vi "load pid.vi"(8 "error in (no error)":errorcluster, 11 "main ref":T1) -> (0 "error out":errorcluster)   [LabVIEW 2025]
uses:
  controls/LAB-IQ UI Data.ctl
  <vilib>/Analysis/baseanly.llb/Mean (DBL).vi
  <vilib>/Utility/error.llb/Trim Whitespace One-Sided.vi
  Instance           5 16Saved   load pid .vi
  <vilib>/Analysis/NI_AALBase.lvlib
  <vilib>/addons/control/pid/NI_PID_autopid.lvlib
panel:
  in  "WriteCC1":string[](array[string])=[""]
  out "apply load 2":bool
  out "Load":dbl
  out "Load Feedback":dbl
  out "Set Load 2":dbl=455.0
  out "Motorised Loading Loop":i32
  out "Zload":dbl
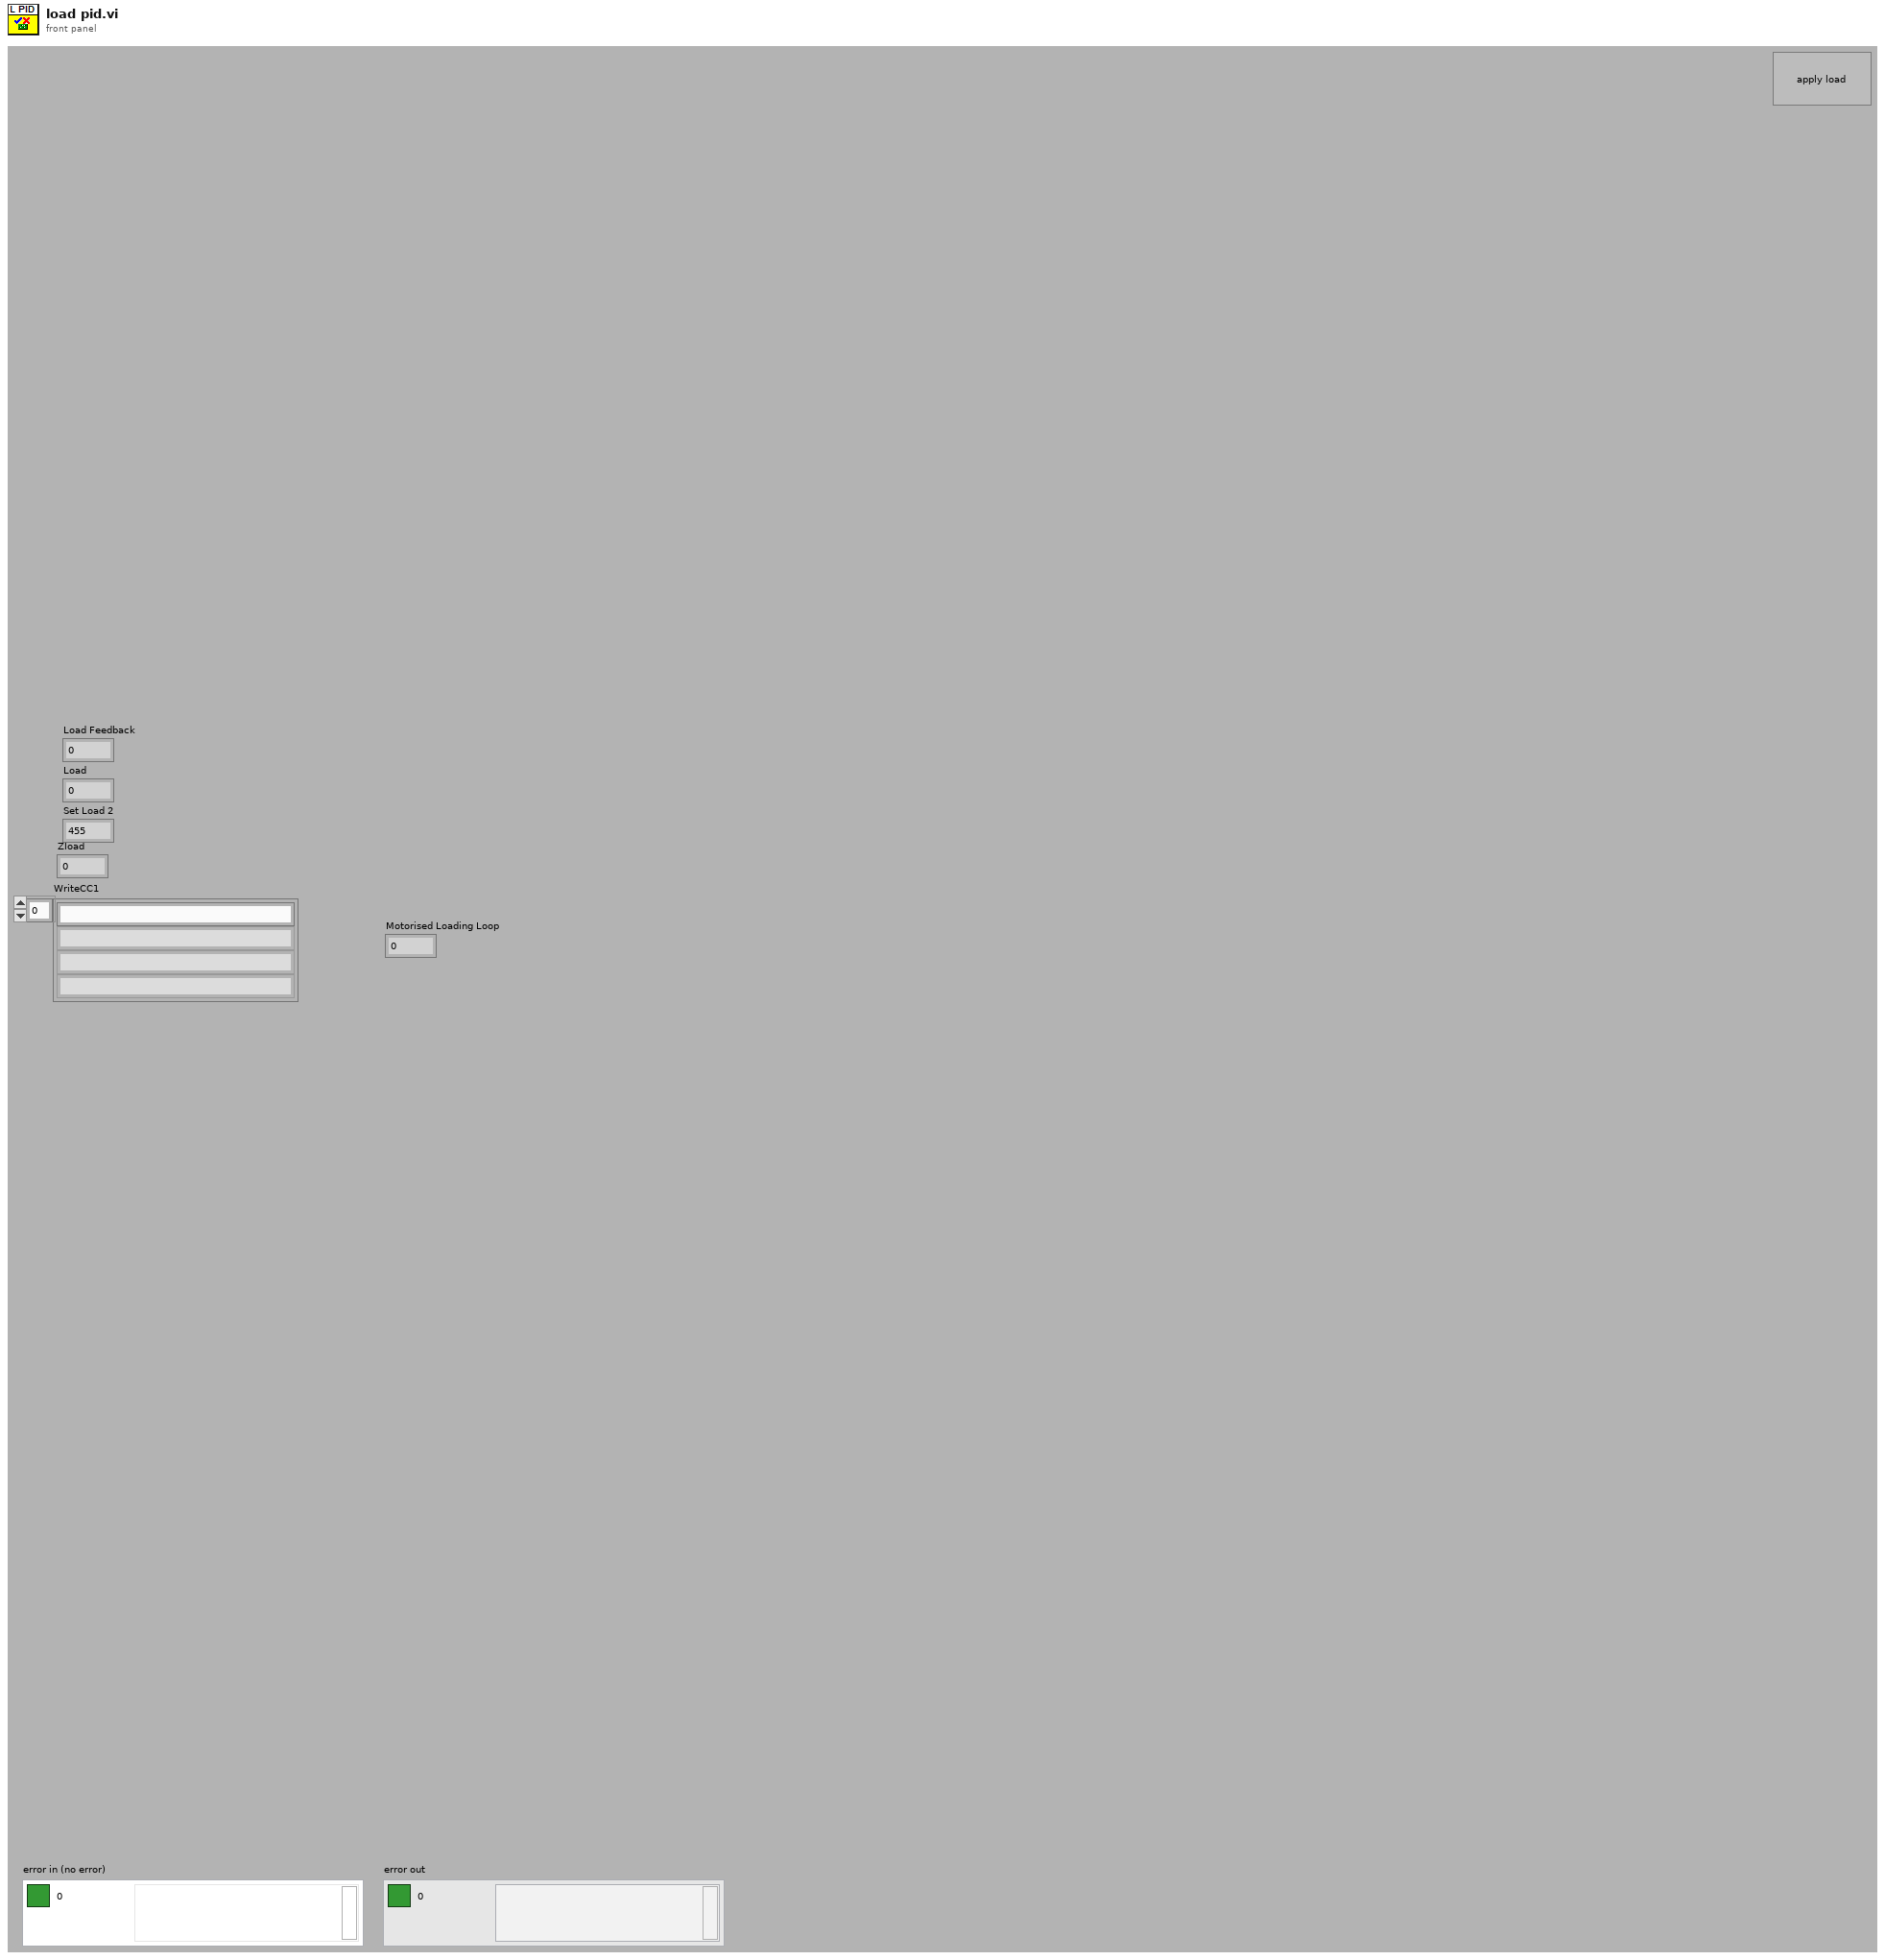
[diagram p1: front panel]
types:
  T1 = typedef "LAB-IQ UI Data.ctl" = cluster{"Main Home Screen":cluster{"GUI":refnum<vi>, "Platform Settings":refnum<vi>, "Configure":refnum<vi>, "Home":refnum<vi>, "EXIT":refnum<vi>, "service 2":refnum<vi>, "MainPage":refnum<vi>, "Analysis":refnum<vi>}, "Platform Settings":cluster{"mm/s  Surge":refnum<vi>, "Update Surge Speed":refnum<vi>, "Drive Error":refnum<vi>, "Disable Axis Jog Soft Limits":refnum<vi>, "mm/s  Sway":refnum<vi>, "Sway and Surge COM Status":refnum<vi>, "Heave COM Status":refnum<vi>, "Enable Platform":refnum<vi>, "Surge Forward Main":refnum<vi>, "Sway Right Main":refnum<vi>, "Sway Left Main":refnum<vi>, "Heave Down Main":refnum<vi>, "Heave Up main":refnum<vi>, "Update Sway Speed":refnum<vi>, "Update Heave Speed":refnum<vi>, "mm/s Heave":refnum<vi>, "mm/sec":refnum<vi>, "mm":refnum<vi>, "Surge Backward Main":refnum<vi>}, "Analysis Screen":cluster{"Analysis Home":refnum<vi>, "Surface Analysis":refnum<vi>, "Imaging":refnum<vi>, "Image Analysis":refnum<vi>, "Post Analysis":refnum<vi>}, "Config Screen":cluster{"Select Load Head":refnum<vi>, "Notes :":refnum<vi>, "FILE":refnum<vi>, "Sample ID :":refnum<vi>, "Operator ID :":refnum<vi>, "Operator Name :":refnum<vi>, "Auto":refnum<vi>}, "Motion Module":cluster{"zNL":refnum<vi>, "NL disp":refnum<vi>, "Rotary Tab":refnum<vi>, "Motion Direction:  3":refnum<vi>, "E.Velocity 2":refnum<vi>, "e.v/ssr 2":refnum<vi>, "Enter Fixed E.Velocity 2":refnum<vi>, "Enter Final SRR 2":refnum<vi>, "Enter initial SRR 2":refnum<vi>, "Enter Fixed SRR 2":refnum<vi>, "Enter the Final E.Velocity (m/s) 2":refnum<vi>, "Enter initial E.Velocity (m/s) 2":refnum<vi>, "Final Speed (RPM) 3":refnum<vi>, "Initial Speed (RPM) 2":refnum<vi>, "Enter the Final Velocity (m/s) 3":refnum<vi>, "Enter initial Velocity (m/s)  3":refnum<vi>, "Ramp Up 2":refnum<vi>, "TEST SELECTION":refnum<vi>, "SPEED SELECTION : ":refnum<vi>, "Angular Oscillation Set":refnum<vi>, "Traction":refnum<vi>, "Step Speed":refnum<vi>, "StepTable For Load-Speed":refnum<vi>, "StepTable For Speed":refnum<vi>, "Surge Forward MM":refnum<vi>, "Surge Backward MM":refnum<vi>, "M3 Image":refnum<vi>, "String 39":refnum<vi>, "Sway Left MM":refnum<vi>, "Sway Right MM":refnum<vi>, "Disable Axis Jog Soft Limits":refnum<vi>, "mm":refnum<vi>, "Heave Down MM":refnum<vi>, "Heave Up MM":refnum<vi>, "Wear Track Diameter (mm)":refnum<vi>, "Set WTD":refnum<vi>, "HomeScratch":refnum<vi>, "HomeRot":refnum<vi>, "PlaceModule":refnum<vi>, "Enter the Angle (Deg)":refnum<vi>, "Enter the Frequency (Hz)":refnum<vi>, "Motion Mode:":refnum<vi>, "LR Sway":refnum<vi>, "Rot Hor":refnum<vi>, "Scratch":refnum<vi>, "LR Cam":refnum<vi>, "MMBack":refnum<vi>, "MMNext":refnum<vi>, "Rot Ver":refnum<vi>, "Rotary Module Selection":refnum<vi>, "calculate rotary":refnum<vi>, "SPEED SELECTION : rotary":refnum<vi>, "Import 2":refnum<vi>, "Save 2":refnum<vi>, "File Path :  2":refnum<vi>, "String 45":refnum<vi>, "StepTable For Speed 3":refnum<vi>, "Enter the Speed(mm/sec)":refnum<vi>, "Enter the Speed(RPM)":refnum<vi>, "Enter Scratch Speed (mm/s):":refnum<vi>, "SwaySpeed Set":refnum<vi>, "Scartch Offset":refnum<vi>, "Motion type:":refnum<vi>, "HomeScratch 2":refnum<vi>, "Enter Scratch length (mm):":refnum<vi>, "Wear Track Diameter":refnum<vi>, "Rotary Speed Exced":refnum<vi>, "Scratch Mode":refnum<vi>, "No of Scratch":refnum<vi>}, "Environmental control":cluster{"Humidity  Status  3":refnum<vi>, "Low Temp  Status  2":refnum<vi>, "TK4 status 2":refnum<vi>, "Stage Temperature":refnum<vi>, "Sample Temperature":refnum<vi>, "Humidity (Amb)":refnum<vi>, "Clear List":refnum<vi>, "Add to list":refnum<vi>, "Wear":refnum<vi>, "Vibration":refnum<vi>, "Humidity (Chamber)":refnum<vi>, "Temperature (Chamber)":refnum<vi>, "ECR ":refnum<vi>, "Temperature (Amb)":refnum<vi>, "Microphone":refnum<vi>, "Acoustic Emission 3":refnum<vi>, "SNext":refnum<vi>, "APBack":refnum<vi>, "Enter the Temperature (°C):":refnum<vi>, "Enter the Stage \nTemperature (°C):":refnum<vi>, "Enter the Humidity (%Rh):":refnum<vi>, "Low Temp":refnum<vi>, "High Temp":refnum<vi>, "Humidity":refnum<vi>, "Sensors Picked":refnum<vi>}, "About Screen":cluster{"Password":refnum<vi>, "Home Service":refnum<vi>, "Advanced Setting":refnum<vi>, "About Tab":refnum<vi>, "ECR Port:":refnum<vi>, "Ramp Port:":refnum<vi>, "Installation/Replacement completed":refnum<vi>, "Loahead":refnum<vi>, "Heave and Surge COM Port:":refnum<vi>, "Sway COM Port:":refnum<vi>, "Temp Modbus:":refnum<vi>, "Humidity Port:":refnum<vi>, "Edit Gain Constants":refnum<vi>, "Save Gain Constants":refnum<vi>}, "Main Screen":cluster{"Main Screen Tab":refnum<vi>, "Angle and Frequency":refnum<vi>, "Stroke (mm)":refnum<vi>, "Angle (Deg)":refnum<vi>, "Main Speed Tab":refnum<vi>, "MTM MOTOR DISPLAY":refnum<vi>, "Disc Speed (m/sec)":refnum<vi>, "Ball Speed (m/sec)":refnum<vi>, "Disc Speed (RPM)":refnum<vi>, "Ball Speed (RPM)":refnum<vi>, "SPEED TAB":refnum<vi>, "Speed (m/sec)":refnum<vi>, "Set Speed (m/sec)":refnum<vi>, "Speed (RPM)":refnum<vi>, "Set Speed":refnum<vi>, "Time Tab":refnum<vi>, "Time ( HH:MM:SS ) 2":refnum<vi>, "Test Duration":refnum<vi>, "Test Duration 4":refnum<vi>, "TEST CYCLE":refnum<vi>, "TOTAL CYCLES":refnum<vi>, "Set Load (N)":refnum<vi>, "Temp Tabs":refnum<vi>, "Heater":refnum<vi>, "TK4 status":refnum<vi>, "ChamberTemp":refnum<vi>, "SetTmp":refnum<vi>, "Controller  Status":refnum<vi>, "ChamberTemp 2":refnum<vi>, "SetTmp 2":refnum<vi>, "Controller  Status 2":refnum<vi>, "ChamberTemp 3":refnum<vi>, "SetTmp 3":refnum<vi>, "Cooling":refnum<vi>, "Load Communication":refnum<vi>, "Ambient \nTemperature":refnum<vi>, "HumCOMStatus":refnum<vi>, "Ambient\n Humidity":refnum<vi>, "Freq (Hz)":refnum<vi>, "Load En":refnum<vi>, "NLt":refnum<vi>, "zNL 2":refnum<vi>, "Humidity On":refnum<vi>, "humidity disp":refnum<vi>, "Set Humidity":refnum<vi>, "NL disp 2":refnum<vi>, "Humidity On 2":refnum<vi>, "humidity disp 2":refnum<vi>, "Set Humidity 2":refnum<vi>, "NL disp 3":refnum<vi>, "AppLoadSeq scratch":refnum<vi>, "Stop Scratch":refnum<vi>, "ClrLog":refnum<vi>, "Trip Log":refnum<vi>, "STOP":refnum<vi>, "Start Test":refnum<vi>, "Test status":refnum<vi>, "AR Led":refnum<vi>, "Data":refnum<vi>, "Health":refnum<vi>, "Sway COM Status":refnum<vi>, "Heave COM Status":refnum<vi>, "Grp Tab":refnum<vi>, "Sub Graph":refnum<vi>, "SD (mm)":refnum<vi>, "Siliding distance Reset Graph":refnum<vi>, "SDGp":refnum<vi>, "Humidity Reset Graph":refnum<vi>, "HumrGp":refnum<vi>, "Acoustic Emission (mV)":refnum<vi>, "Aqucostic Reset Graph":refnum<vi>, "gACQUOS":refnum<vi>, "ECR RESET":refnum<vi>, "ECR":refnum<vi>, "Temperature Reset":refnum<vi>, "Acoustic Emission (mV) 2":refnum<vi>, "Aqucostic Reset Graph 2":refnum<vi>, "gACQUOS 2":refnum<vi>, "ECR RESET 2":refnum<vi>, "ECR 2":refnum<vi>, "Temperature Reset 2":refnum<vi>, "Temperature (deg c)":refnum<vi>, "Speed Reset Graph":refnum<vi>, "Speed Tab":refnum<vi>, "MTM DISC  SPEED":refnum<vi>, "MTM BALL SPEED":refnum<vi>, "speed mm/sec":refnum<vi>, "Hymidity":refnum<vi>, "Humidity Disable trip":refnum<vi>, "CoF Trip  2":refnum<vi>, "Depth Trip":refnum<vi>, "Weart Deapth":refnum<vi>, "Depth Reset Graph":refnum<vi>, "Weart":refnum<vi>, "Depthz":refnum<vi>, "Depth (µm)":refnum<vi>, "WearGp":refnum<vi>, "NL Trip 2":refnum<vi>, "Load pid":refnum<vi>, "Load Disable Trip":refnum<vi>, "Load Reset Graph":refnum<vi>, "NL Display 4":refnum<vi>, "Main Chart 3":refnum<vi>, "BACK":refnum<vi>, "Depth Trip 2":refnum<vi>, "COF TRIP ":refnum<vi>, "Friction Force (N)":refnum<vi>, "FF Reset Graph":refnum<vi>, "FF Disable Trip":refnum<vi>, "FF TRIP":refnum<vi>, "COF Disable Trip":refnum<vi>, "COF Reset Graph":refnum<vi>, "Start Test Temp":refnum<vi>, "zFF":refnum<vi>, "Friction Force (N) Graph":refnum<vi>, "Coefficient of Friction":refnum<vi>, "Scratch Start Test":refnum<vi>, "FF Tab":refnum<vi>, "Cyclic Friction Force (N)":refnum<vi>, "CZ FF":refnum<vi>, "Cyclic Friction Force (N) Graph":refnum<vi>, "Cyclic Coefficient of Friction":refnum<vi>, "Cyclic FF TRIP":refnum<vi>, "Cyclic FF Disable Trip":refnum<vi>, "cyclic COF Disable Trip":refnum<vi>, "cyclic COF TRIP":refnum<vi>, "cyclic COF Reset Graph":refnum<vi>, "Cyclic FF Reset Graph":refnum<vi>, "Test Trip":refnum<vi>, "Multi Scratch Pass":refnum<vi>}, "Loading":cluster{"Indentation":refnum<vi>, "Reference Sample":refnum<vi>, "Load Cell Communication Slide":refnum<vi>, "com 3":refnum<vi>, "com":refnum<vi>, "DecaForce COM Status":refnum<vi>, "Update":refnum<vi>, "Clear 3":refnum<vi>, "seq":refnum<vi>, "Stribeck table":refnum<vi>, "Stribeck Table  For loading":refnum<vi>, "Loading Mode":refnum<vi>, "Enter the Final Load (N)":refnum<vi>, "Enter the CoF Trip":refnum<vi>, "Enter the Friction Force Trip":refnum<vi>, "Enter the Normal load Trip":refnum<vi>, "Enter the Load  (N)":refnum<vi>, "KiloForce":refnum<vi>, "DecaForce ":refnum<vi>, "MicroForce":refnum<vi>, "LHBack":refnum<vi>, "LHNext":refnum<vi>, "Enter the Loading Rate (N/min)":refnum<vi>, "Message":refnum<vi>, "Warning 2":refnum<vi>, "SSP 0.75":refnum<vi>, "SSP 0.5":refnum<vi>, "SSP 0.3":refnum<vi>, "Warning":refnum<vi>, "gui GIF":refnum<vi>, "Communication is established":refnum<vi>, "AppLoad 4":refnum<vi>, "Multipoint":refnum<vi>, "Load Selection":refnum<vi>}, "PID":cluster{"Ramp MulFac":refnum<vi>, "pulses LoadDiffRamp(2..10)":refnum<vi>, "PulseControlRamp(diff<=3N)":refnum<vi>, "SetLoadDeadband(%) Load(0-10N)":refnum<vi>, "PID gains out delay (microForce)":refnum<vi>, "Ramp":refnum<vi>, "Gain 2":refnum<vi>, "pulses LoadDiff(2..10)":refnum<vi>, "pulses LoadDiff(11..50)":refnum<vi>, "PulseControl(diff<=3N)":refnum<vi>, "SetLoadDeadband(%)  2":refnum<vi>, "Dummy Run":refnum<vi>, "Vertical load (N)":refnum<vi>, "AutoTune":refnum<vi>, "Offset 3 ":refnum<vi>, "apply load":refnum<vi>, "Offset  3":refnum<vi>, "apply load 2":refnum<vi>, "Enter ByPass Load":refnum<vi>, "reinit 3":refnum<vi>, "output range delay":refnum<vi>, "PID gains out delay":refnum<vi>, "Bypass Load":refnum<vi>, "pulsesSent":refnum<vi>, "pulses ":refnum<vi>, "actpid":refnum<vi>, "gFF Rot":refnum<vi>, "pulses LoadDiff(21..1000)":refnum<vi>, "Delay":refnum<vi>, "deadband":refnum<vi>}, "Config Parameters":cluster{"Tab Control 3":refnum<vi>, "Tab Control 19":refnum<vi>, "SAMPLES":refnum<vi>, "Re-initilaize":refnum<vi>, "Filter ON/OFF":refnum<vi>, "TracHomeSurgeOffsetCounts 10MM":refnum<vi>, "TracHomeSwayOffsetCounts 10MM":refnum<vi>, "Acoustic Emission:":refnum<vi>, "Apply Filter (FF)":refnum<vi>, "Filter% 2":refnum<vi>, "Apply Filter (Load)":refnum<vi>, "Filter% ":refnum<vi>, "Sway distance (mm)":refnum<vi>, "Surge distance (mm)":refnum<vi>, "DataSavingLoopDelay(ms)":refnum<vi>, "SAVE 2":refnum<vi>, "Enter Distance":refnum<vi>, "Sway Counts:":refnum<vi>, "Distance (mm): 3":refnum<vi>, "Surge Counts:":refnum<vi>, "Distance (mm): 2":refnum<vi>, "Distance (mm):":refnum<vi>, "Heave Counts:":refnum<vi>, "LRMHomeSurgeOffsetCounts":refnum<vi>, "LRMHomeSwayOffsetCounts":refnum<vi>, "TracHomeSurgeOffsetCounts 20MM":refnum<vi>, "TracHomeSwayOffsetCounts 20MM":refnum<vi>, "RotHomeSwayOffsetCounts":refnum<vi>, "RotHomeSurgeOffsetCounts":refnum<vi>, "Heave distance":refnum<vi>, "Zmm":refnum<vi>, "Heave Pulses/mm":refnum<vi>, "Surge Pulses/mm":refnum<vi>, "Sway Pulses/mm":refnum<vi>, "Heave Pitch":refnum<vi>, "Surge Pitch":refnum<vi>, "Sway Pitch":refnum<vi>, "Heave PPR":refnum<vi>, "Surge PPR":refnum<vi>, "Sway PPR":refnum<vi>, "Tab Control 5":refnum<vi>, "Tab Control 14":refnum<vi>, "Tab Control 26":refnum<vi>, "AE":refnum<vi>, "Heave Loop Delay":refnum<vi>, "Heave PID Speed":refnum<vi>, "Surge Jog Speed":refnum<vi>, "Heave Jog Speed":refnum<vi>, "Sway Loop Delay":refnum<vi>, "Sway PID Speed":refnum<vi>, "Sway Jog Speed":refnum<vi>}, "Loading Com Port":cluster{"ClearAll":refnum<vi>, "Mz(Nm)":refnum<vi>, "My(Nm)":refnum<vi>, "Mx(Nm)":refnum<vi>, "Save Dwell":refnum<vi>, "Mx ":refnum<vi>, "My ":refnum<vi>, "Mz":refnum<vi>, "Fx(N)":refnum<vi>, "Fy(N)":refnum<vi>, "Fz(N)":refnum<vi>, "ZeroAll":refnum<vi>, "Acq Delay (ms)":refnum<vi>, "Burst Delay (ms)":refnum<vi>, "model":refnum<vi>, "SN":refnum<vi>, "FFx(N)":refnum<vi>, "Sensor IP":refnum<vi>, "Port":refnum<vi>, "FFy(N)":refnum<vi>, "Load(N)":refnum<vi>, "delete Handle":refnum<vi>, "Create Handle":refnum<vi>, "ft_data":refnum<vi>, "ft_range":refnum<vi>, "ft_data 2":refnum<vi>, "stop 6":refnum<vi>, "running_flag":refnum<vi>, "ft_udp_handle":refnum<vi>, "get-data-return":refnum<vi>, "get-range-return":refnum<vi>, "zero-return":refnum<vi>, "filter-return":refnum<vi>, "initial-return":refnum<vi>, "deleteHandle-result":refnum<vi>, "Load Cell Temp":refnum<vi>}, "Heave AND Surge":cluster{"SURGE POSE":refnum<vi>, "error out Read":refnum<vi>, "HEAVE POSE":refnum<vi>, "State":refnum<vi>, "Homed":refnum<vi>, "Sequence ID":refnum<vi>, "error out Write":refnum<vi>, "faultCode":refnum<vi>, "Ack ID":refnum<vi>, "SPEED":refnum<vi>, "Distance":refnum<vi>, "Mode Command":refnum<vi>, "Heave and Surge Read":refnum<vi>, "Read Heave Temp":refnum<vi>, "Spare 15":refnum<vi>, "Spare 14":refnum<vi>, "Spare 13":refnum<vi>, "Spare 12":refnum<vi>, "Spare 11":refnum<vi>, "Spare 10":refnum<vi>, "Spare 9":refnum<vi>, "Spare 8":refnum<vi>, "Spare 7":refnum<vi>, "Spare 6":refnum<vi>, "Spare 5":refnum<vi>, "Spare 4":refnum<vi>, "Spare 2":refnum<vi>, "Spare 1":refnum<vi>, "Node Id":refnum<vi>, "Spare 3":refnum<vi>, "SPARE 4":refnum<vi>, "SPARE 3":refnum<vi>, "SPARE 2":refnum<vi>, "SPARE 1":refnum<vi>, "fwMajor":refnum<vi>, "fwMinor":refnum<vi>, "Manual Write":refnum<vi>, "Heave and Surge Write":refnum<vi>}, "New PID LOGIC":cluster{"Fine Tune Zone":refnum<vi>, "PID SDelay":refnum<vi>, "Max_pos_limit":refnum<vi>, "Min_pos_limit":refnum<vi>, "i_limit":refnum<vi>, "pct_scale":refnum<vi>, "Deadband":refnum<vi>, "Kd":refnum<vi>, "Ki":refnum<vi>, "Kp":refnum<vi>, "Current Position":refnum<vi>, "Set Load":refnum<vi>, "Current Load":refnum<vi>, "Pulse delta":refnum<vi>, "Init Step":refnum<vi>, "Max Step Linit":refnum<vi>}, "SWAY ":cluster{"fwMajor":refnum<vi>, "Homed":refnum<vi>, "Rotary POSE":refnum<vi>, "State":refnum<vi>, "SWAY POSE":refnum<vi>, "Ack ID":refnum<vi>, "faultCode":refnum<vi>, "Node Id":refnum<vi>, "fwMinor":refnum<vi>, "Spare 6":refnum<vi>, "Spare 5":refnum<vi>, "Spare 4":refnum<vi>, "Spare 3":refnum<vi>, "Spare 2":refnum<vi>, "Spare 1":refnum<vi>, "Spare 7":refnum<vi>, "SPARE  5":refnum<vi>, "error out Write  SWAY ":refnum<vi>, "error out Read SWAY ":refnum<vi>, "Manual Write SWAY ":refnum<vi>, "SWAY WRITE":refnum<vi>, "SPARE  4":refnum<vi>, "SPARE  3":refnum<vi>, "SPARE 2":refnum<vi>, "SPARE 1":refnum<vi>, "Spare 15":refnum<vi>, "Spare 14":refnum<vi>, "Spare 13":refnum<vi>, "Spare 12":refnum<vi>, "Spare 11":refnum<vi>, "Spare 9":refnum<vi>, "Spare 8":refnum<vi>, "SPEED":refnum<vi>, "Distance":refnum<vi>, "Mode Command":refnum<vi>, "Sequence ID":refnum<vi>, "SWAY READ":refnum<vi>, "Spare 10":refnum<vi>, "Read SWAY Temp":refnum<vi>}, "Analysis Screen":cluster{"Analysis Home":refnum<vi>, "Refresh 2":refnum<vi>, "MEAN 4":refnum<vi>, "SD 4":refnum<vi>, "VARIANCE 4":refnum<vi>, "MEAN  3":refnum<vi>, "SD  3":refnum<vi>, "VARIANCE  3":refnum<vi>, "MEAN 2":refnum<vi>, "SD  2":refnum<vi>, "VARIANCE 2":refnum<vi>, "MEAN":refnum<vi>, "SD":refnum<vi>, "VARIANCE":refnum<vi>, "File 4 Discription":refnum<vi>, "OPEN 4":refnum<vi>, "File Name 4":refnum<vi>, "OPEN 3":refnum<vi>, "File 3 Discription":refnum<vi>, "File Name 3":refnum<vi>, "Y-AXIS":refnum<vi>, "X-AXIS":refnum<vi>, "XY Graph":refnum<vi>, "File Name 2":refnum<vi>, "File Name 1":refnum<vi>, "OPEN 2":refnum<vi>, "OPEN 1":refnum<vi>, "File 1 Discription ":refnum<vi>, "File 2 Discription":refnum<vi>}}
  T2 = enum8{"Enabled", "Disabled", "Disabled and Grayed Out"}
  T3 = cluster{"proportional gain (Kc)":dbl, "integral time (Ti, min)":dbl, "derivative time (Td, min)":dbl}
  T4 = cluster{"Value":dbl, "Load Feedback":dbl, "output":dbl}
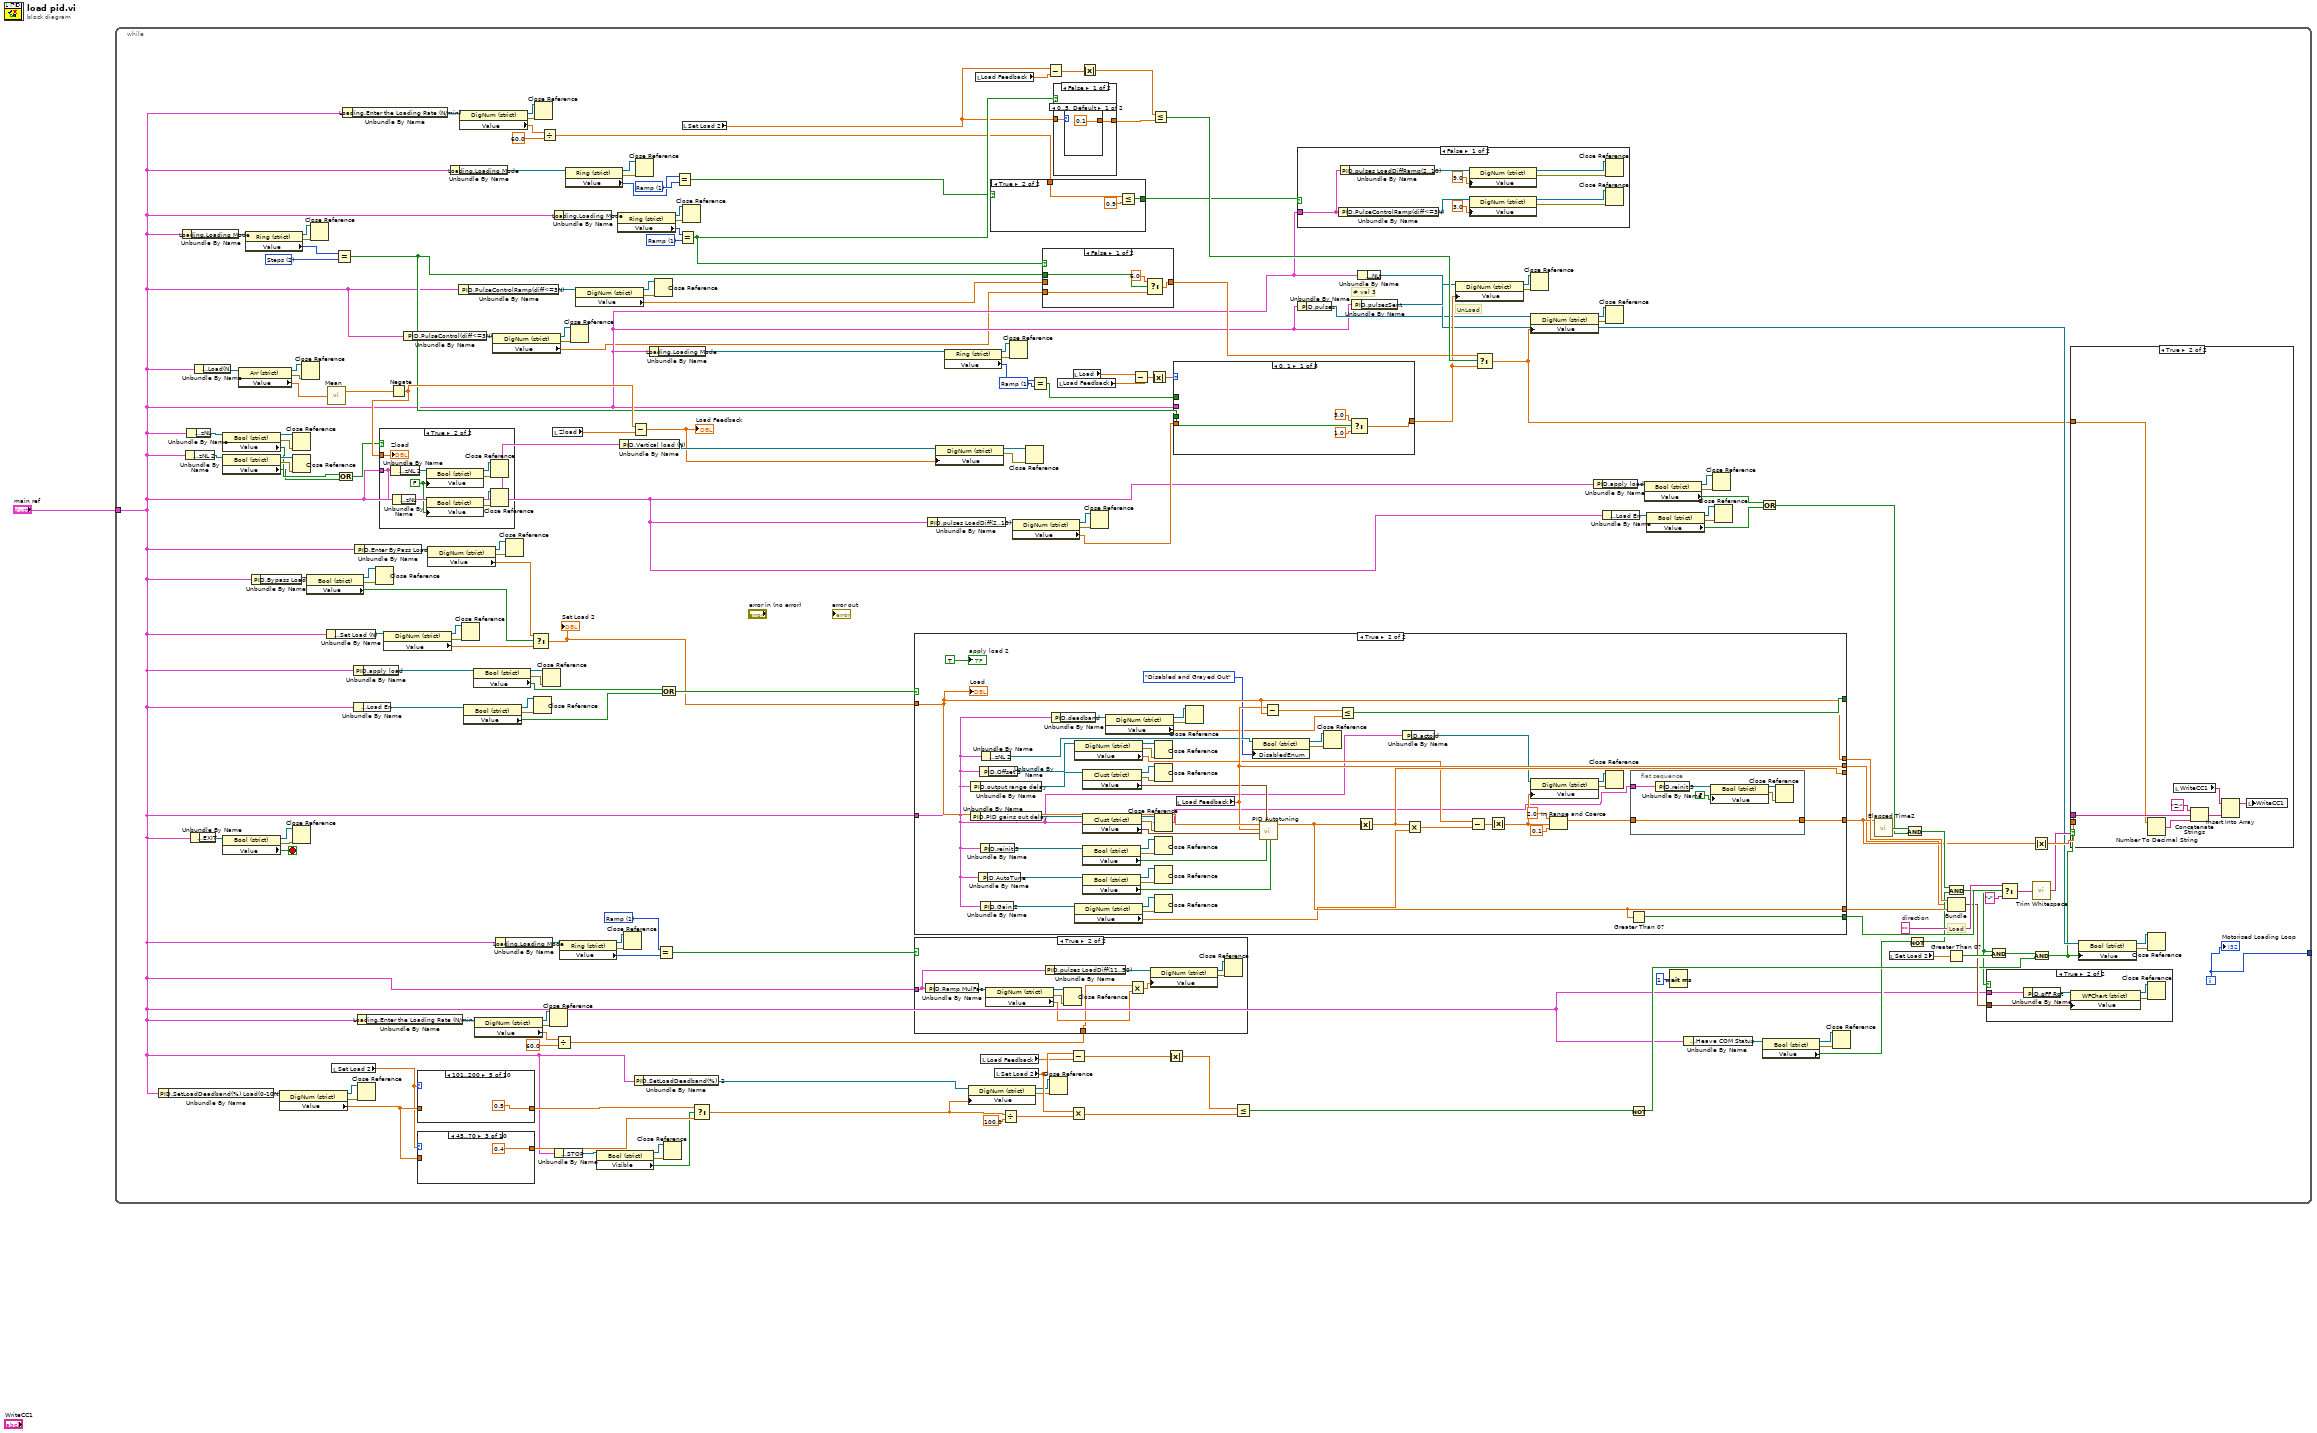
[diagram p0: block diagram]
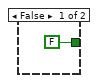
[diagram p2: hidden frame]
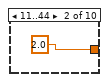
[diagram p4: hidden frame]
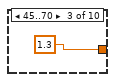
[diagram p5: hidden frame]
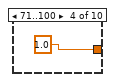
[diagram p6: hidden frame]
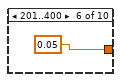
[diagram p7: hidden frame]
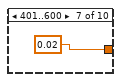
[diagram p8: hidden frame]
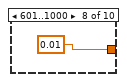
[diagram p9: hidden frame]
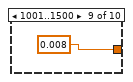
[diagram p10: hidden frame]
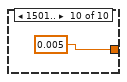
[diagram p11: hidden frame]
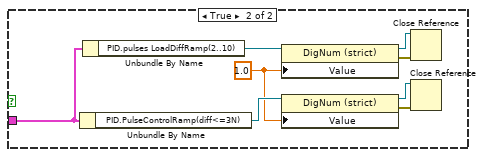
[diagram p12: hidden frame]
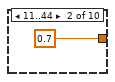
[diagram p15: hidden frame]
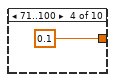
[diagram p16: hidden frame]
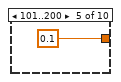
[diagram p17: hidden frame]
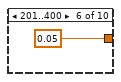
[diagram p18: hidden frame]
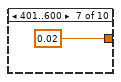
[diagram p19: hidden frame]
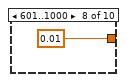
[diagram p20: hidden frame]
diagram:
  n1 = while {
    tunnel: [w156] -> _
    tunnel: "main ref" -> [w4]
    i -> [w156]
    stop <- w122 stop-if-true
    w37 = u16 1 items=["Constant", "Ramp", "Steps", "Indentation"] ("Loading Mode")
    w128 = u16 1 items=["Constant", "Ramp", "Steps", "Indentation"] ("Loading Mode")
    w130 = u16 2 items=["Constant", "Ramp", "Steps", "Indentation"] ("Loading Mode")
    w141 = u16 1 items=["Constant", "Ramp", "Steps", "Indentation"] ("Loading Mode")
    w143 = u16 1 items=["Constant", "Ramp", "Steps", "Indentation"] ("Loading Mode")
    w182 = ""  # direction
    # "# val 3"
    # "UnLoad"
    # "Load"
    n2 = Unbundle By Name(w4) -> ("PID.SetLoadDeadband(%) Load(0-10N)"=w68:refnum<vi>)
    n3 = Unbundle By Name(w4) -> ("Loading.Loading Mode"=w33:refnum<vi>)
    n4 = Unbundle By Name(w4) -> ("Main Screen.zNL 2"=w108:refnum<vi>)
    n5 = Unbundle By Name(w4) -> ("Motion Module.zNL"=w113:refnum<vi>)
    n6 = Unbundle By Name(w4) -> ("Main Home Screen.EXIT"=w125:refnum<vi>)
    n7 = Unbundle By Name(w4) -> ("Loading Com Port.Load(N)"=w115:refnum<vi>)
    n8 = property class="Bool (strict)"(reference=w113) -> (reference out=w111:refnum<vi>, error out=w112:errorcluster, "Value"=w107:bool)  [unwired: 1 in]
    n9 = property class="Bool (strict)"(reference=w108) -> (reference out=w110:refnum<vi>, error out=w109:errorcluster, "Value"=w106:bool)  [unwired: 1 in]
    n10 = property class="Bool (strict)"(reference=w125) -> (reference out=w123:refnum<vi>, error out=w124:errorcluster, "Value"=w122:bool)  [unwired: 1 in]
    n11 = property class="Arr (strict)"(reference=w115) -> (reference out=w117:refnum<vi>, error out=w116:errorcluster, "Value"=w114:dbl[])  [unwired: 1 in]
    n12 = property class="Ring (strict)"(reference=w33) -> (reference out=w32:refnum<vi>, error out=w34:errorcluster, "Value"=w31:u16)  [unwired: 1 in]
    n13 = Unbundle By Name(w4) -> ("PID.Bypass Load"=w77:refnum<vi>)
    n14 = property class="DigNum (strict)"(reference=w68) -> (reference out=w70:refnum<vi>, error out=w69:errorcluster, "Value"=w67:dbl)  [unwired: 1 in]
    n15 = Close Reference(reference=w111, error in (no error)=w112) -> ()  [unwired: 1 out]
    n16 = Close Reference(reference=w110, error in (no error)=w109) -> ()  [unwired: 1 out]
    n17 = Close Reference(reference=w123, error in (no error)=w124) -> ()  [unwired: 1 out]
    n18 = Close Reference(reference=w117, error in (no error)=w116) -> ()  [unwired: 1 out]
    n19 = property class="Bool (strict)"(reference=w77) -> (reference out=w75:refnum<vi>, error out=w76:errorcluster, "Value"=w74:bool)  [unwired: 1 in]
    n20 = Close Reference(reference=w32, error in (no error)=w34) -> ()  [unwired: 1 out]
    n21 = Unbundle By Name(w4) -> ("Main Screen.Set Load (N)"=w80:refnum<vi>)
    n22 = call-poly <vilib>:"Mean.vi"("X"=w114) -> ("mean"=w146:dbl)  [unwired: 1 out]
    n23 = local read "Set Load 2"() -> (w41:dbl)
    n24 = Equal?(x=w31, y=w130) -> (x = y?=w129:bool)
    n25 = Or(x=w107, y=w106) -> (x .or. y?=w126:bool)
    n26 = Unbundle By Name(w4) -> ("Loading.Enter the Loading Rate (N/min)"=w14:refnum<vi>)
    n27 = Unbundle By Name(w4) -> ("PID.apply load"=w95:refnum<vi>)
    n28 = Unbundle By Name(w4) -> ("Main Screen.Load En"=w101:refnum<vi>)
    n29 = Unbundle By Name(w4) -> ("PID.Enter ByPass Load"=w85:refnum<vi>)
    n30 = Unbundle By Name(w4) -> ("Loading.Enter the Loading Rate (N/min)"=w20:refnum<vi>)
    n31 = Close Reference(reference=w70, error in (no error)=w69) -> ()  [unwired: 1 out]
    n32 = Close Reference(reference=w75, error in (no error)=w76) -> ()  [unwired: 1 out]
    n33 = property class="DigNum (strict)"(reference=w80) -> (reference out=w82:refnum<vi>, error out=w81:errorcluster, "Value"=w78:dbl)  [unwired: 1 in]
    n34 = Negate(x=w146) -> (-x=w140:dbl)
    n35 = case shown="True" w126 {
      tunnel: w140 -> [_ w261]
      tunnel: w4 -> [_ w254]
      frame False {
      }
      frame True {
        w253 = FALSE ("Value")
        n36 = Unbundle By Name(w254) -> ("Main Screen.zNL 2"=w260:refnum<vi>)
        n37 = Unbundle By Name(w254) -> ("Motion Module.zNL"=w255:refnum<vi>)
        n38 = property class="Bool (strict)"(reference=w260, "Value"=w253) -> (reference out=w258:refnum<vi>, error out=w259:errorcluster)  [unwired: 1 in]
        n39 = property class="Bool (strict)"(reference=w255, "Value"=w253) -> (reference out=w257:refnum<vi>, error out=w256:errorcluster)  [unwired: 1 in]
        n40 = Close Reference(reference=w258, error in (no error)=w259) -> ()  [unwired: 1 out]
        n41 = Close Reference(reference=w257, error in (no error)=w256) -> ()  [unwired: 1 out]
        "Zload" <- w261
      }
    }
    n42 = Unbundle By Name(w4) -> ("PID.PulseControl(diff<=3N)"=w6:refnum<vi>)
    n43 = case shown="101..200" w41 {
      tunnel: [w188 2.0 ("y") 1.3 ("y") 1.0 ("y") 0.5 ("y") 0.05 ("y") 0.02 ("y") 0.01 ("y") 0.008 ("y") 0.005 ("y")] -> w132
      tunnel: w67 -> [w188 _ _ _ _ _ _ _ _ _]
      frame 0..10, Default {
      }
      frame 11..44 {
      }
      frame 45..70 {
      }
      frame 71..100 {
      }
      frame 101..200 {
      }
      frame 201..400 {
      }
      frame 401..600 {
      }
      frame 601..1000 {
      }
      frame 1001..1500 {
      }
      frame 1501.. {
      }
    }
    n44 = case shown="45..70" w41 {
      tunnel: [w220 0.7 ("y") 0.4 ("y") 0.1 ("y") 0.1 ("y") 0.05 ("y") 0.02 ("y") 0.01 ("y") 0.008 ("y") 0.005 ("y")] -> w131
      tunnel: w67 -> [w220 _ _ _ _ _ _ _ _ _]
      frame 0..10, Default {
      }
      frame 11..44 {
      }
      frame 45..70 {
      }
      frame 71..100 {
      }
      frame 101..200 {
      }
      frame 201..400 {
      }
      frame 401..600 {
      }
      frame 601..1000 {
      }
      frame 1001..1500 {
      }
      frame 1501.. {
      }
    }
    n45 = property class="DigNum (strict)"(reference=w85) -> (reference out=w83:refnum<vi>, error out=w84:errorcluster, "Value"=w79:dbl)  [unwired: 1 in]
    n46 = Unbundle By Name(w4) -> ("Loading.Loading Mode"=w121:refnum<vi>)
    n47 = Unbundle By Name(w4) -> ("PID.PulseControlRamp(diff<=3N)"=w47:refnum<vi>)
    n48 = property class="DigNum (strict)"(reference=w14) -> (reference out=w16:refnum<vi>, error out=w15:errorcluster, "Value"=w13:dbl)  [unwired: 1 in]
    n49 = Close Reference(reference=w82, error in (no error)=w81) -> ()  [unwired: 1 out]
    n50 = property class="Bool (strict)"(reference=w101) -> (reference out=w99:refnum<vi>, error out=w100:errorcluster, "Value"=w98:bool)  [unwired: 1 in]
    n51 = property class="Bool (strict)"(reference=w95) -> (reference out=w97:refnum<vi>, error out=w96:errorcluster, "Value"=w94:bool)  [unwired: 1 in]
    n52 = property class="DigNum (strict)"(reference=w20) -> (reference out=w22:refnum<vi>, error out=w21:errorcluster, "Value"=w19:dbl)  [unwired: 1 in]
    n53 = property class="DigNum (strict)"(reference=w6) -> (reference out=w3:refnum<vi>, error out=w5:errorcluster, "Value"=w2:dbl)  [unwired: 1 in]
    n54 = Unbundle By Name(w4) -> ("Loading.Loading Mode"=w38:refnum<vi>)
    n55 = Close Reference(reference=w83, error in (no error)=w84) -> ()  [unwired: 1 out]
    n56 = Select(t=w79, s=w74, f=w78) -> (s? t:f=w134:dbl)
    "Set Load 2" <- w134
    n57 = Close Reference(reference=w99, error in (no error)=w100) -> ()  [unwired: 1 out]
    n58 = Close Reference(reference=w16, error in (no error)=w15) -> ()  [unwired: 1 out]
    n59 = Divide(x=w13, y=60.0) -> (x/y=w11:dbl)
    n60 = Close Reference(reference=w97, error in (no error)=w96) -> ()  [unwired: 1 out]
    n61 = Close Reference(reference=w22, error in (no error)=w21) -> ()  [unwired: 1 out]
    n62 = local read "Zload"() -> (w145:dbl)
    n63 = Unbundle By Name(w4) -> ("Loading.Loading Mode"=w73:refnum<vi>)
    n64 = Unbundle By Name(w4) -> ("Main Screen.STOP"=w24:refnum<vi>)
    n65 = Divide(x=w19, y=60.0) -> (x/y=w17:dbl)
    n66 = property class="Ring (strict)"(reference=w38) -> (reference out=w40:refnum<vi>, error out=w39:errorcluster, "Value"=w36:u16)  [unwired: 1 in]
    n67 = property class="Ring (strict)"(reference=w121) -> (reference out=w119:refnum<vi>, error out=w120:errorcluster, "Value"=w118:u16)  [unwired: 1 in]
    n68 = Close Reference(reference=w3, error in (no error)=w5) -> ()  [unwired: 1 out]
    n69 = property class="DigNum (strict)"(reference=w47) -> (reference out=w49:refnum<vi>, error out=w48:errorcluster, "Value"=w46:dbl)  [unwired: 1 in]
    n70 = property class="Bool (strict)"(reference=w24) -> (reference out=w26:refnum<vi>, error out=w25:errorcluster, "Visible"=w23:bool)  [unwired: 1 in]
    n71 = property class="Ring (strict)"(reference=w73) -> (reference out=w71:refnum<vi>, error out=w72:errorcluster, "Value"=w66:u16)  [unwired: 1 in]
    n72 = Unbundle By Name(w4) -> ("PID.Vertical load (N)"=w103:refnum<vi>)
    n73 = Close Reference(reference=w40, error in (no error)=w39) -> ()  [unwired: 1 out]
    n74 = Subtract(x=w140, y=w145) -> (x-y=w102:dbl)
    "Load Feedback" <- w102
    n75 = Unbundle By Name(w4) -> ("PID.SetLoadDeadband(%)  2"=w45:refnum<vi>)
    n76 = Close Reference(reference=w119, error in (no error)=w120) -> ()  [unwired: 1 out]
    n77 = Unbundle By Name(w4) -> ("Loading.Loading Mode"=w29:refnum<vi>)
    n78 = Close Reference(reference=w49, error in (no error)=w48) -> ()  [unwired: 1 out]
    n79 = Equal?(x=w37, y=w36) -> (x = y?=w35:bool)
    n80 = Or(x=w94, y=w98) -> (x .or. y?=w179:bool)
    n81 = Close Reference(reference=w26, error in (no error)=w25) -> ()  [unwired: 1 out]
    n82 = Equal?(x=w118, y=w128) -> (x = y?=w127:bool)
    n83 = Equal?(x=w66, y=w143) -> (x = y?=w137:bool)
    n84 = local read "Set Load 2"() -> (w133:dbl)
    n85 = Close Reference(reference=w71, error in (no error)=w72) -> ()  [unwired: 1 out]
    n86 = Select(t=w132, s=w23, f=w131) -> (s? t:f=w42:dbl)
    n87 = case shown="True" w179 {
      tunnel: [w309 w375] -> w154
      tunnel: [_ w373] -> _
      tunnel: [0.0 ("y") w370] -> w159
      tunnel: [w309 w369] -> w138
      tunnel: w134 -> [_ w370]
      tunnel: [_ w368] -> w170
      tunnel: [w307 w367] -> w158
      tunnel: [w307 w366] -> _
      tunnel: w4 -> [w302 w325]
      frame False {
        w307 = 0.0 ("output")
        w309 = 1000.0 ("output")
        n88 = local read "apply load 2"() -> (w308:bool)
        n89 = case shown="True" w308 {
          tunnel: w302 -> [w313 w316]
          frame False {
            n90 = Unbundle By Name(w313) -> ("PID.Bypass Load"=w314:refnum<vi>)
            n91 = property class="Bool (strict)"(reference=w314, "Value"=TRUE ("FLg")) -> (reference out=w311:refnum<vi>, error out=w315:errorcluster)  [unwired: 1 in]
            n92 = Close Reference(reference=w311, error in (no error)=w315) -> ()  [unwired: 1 out]
          }
          frame True {
            n93 = stacked-sequence {
              tunnel: w316 -> [_ _]
              frame #0 {
                n94 = Concatenate Strings("Z;", "-" ("string"), "7466" ("string")) -> (w320:string)
                n95 = local read "WriteCC1"() -> (w322:string[])
                n96 = Insert Into Array(array=w322, new element=w320) -> (w321:string[])  [unwired: 1 in]
                n97 = local write "WriteCC1"(w321) -> ()
              }
              frame #1 {
                n98 = local write "apply load 2"(FALSE ("apply load 2")) -> ()
                n99 = Wait (ms)(milliseconds to wait=u32 1000) -> ()  [unwired: 1 out]
              }
            }
          }
        }
        n100 = Unbundle By Name(w302) -> ("Main Screen.zNL 2"=w306:refnum<vi>)
        n101 = property class="Bool (strict)"(reference=w306, "DisabledEnum"=T2."Enabled" ("Disabled")) -> (reference out=w304:refnum<vi>, error out=w305:errorcluster)  [unwired: 1 in]
        n102 = Close Reference(reference=w304, error in (no error)=w305) -> ()  [unwired: 1 out]
      }
      frame True {
        n103 = Unbundle By Name(w325) -> ("PID.output range delay"=w351:refnum<vi>)
        n104 = Unbundle By Name(w325) -> ("PID.PID gains out delay"=w359:refnum<vi>)
        n105 = Unbundle By Name(w325) -> ("PID.AutoTune"=w342:refnum<vi>)
        n106 = Unbundle By Name(w325) -> ("PID.Offset 3"=w331:refnum<vi>)
        n107 = Unbundle By Name(w325) -> ("PID.reinit 3"=w336:refnum<vi>)
        n108 = Unbundle By Name(w325) -> ("PID.Gain 2"=w345:refnum<vi>)
        n109 = Unbundle By Name(w325) -> ("Main Screen.zNL 2"=w357:refnum<vi>)
        n110 = Unbundle By Name(w325) -> ("PID.deadband"=w347:refnum<vi>)
        n111 = property class="DigNum (strict)"(reference=w331) -> (reference out=w333:refnum<vi>, error out=w332:errorcluster, "Value"=w330:dbl)  [unwired: 1 in]
        n112 = property class="DigNum (strict)"(reference=w345) -> (reference out=w343:refnum<vi>, error out=w344:errorcluster, "Value"=w334:dbl)  [unwired: 1 in]
        n113 = property class="Clust (strict)"(reference=w351) -> (reference out=w353:refnum<vi>, error out=w352:errorcluster, "Value"=w350:cluster{"output high":dbl, "output low":dbl})  [unwired: 1 in]
        n114 = property class="Clust (strict)"(reference=w359) -> (reference out=w361:refnum<vi>, error out=w360:errorcluster, "Value"=w358:T3)  [unwired: 1 in]
        n115 = property class="Bool (strict)"(reference=w336) -> (reference out=w338:refnum<vi>, error out=w337:errorcluster, "Value"=w335:bool)  [unwired: 1 in]
        n116 = property class="Bool (strict)"(reference=w342) -> (reference out=w340:refnum<vi>, error out=w341:errorcluster, "Value"=w339:bool)  [unwired: 1 in]
        n117 = property class="DigNum (strict)"(reference=w347) -> (reference out=w349:refnum<vi>, error out=w348:errorcluster, "Value"=w346:dbl)  [unwired: 1 in]
        n118 = Close Reference(reference=w333, error in (no error)=w332) -> ()  [unwired: 1 out]
        n119 = Close Reference(reference=w353, error in (no error)=w352) -> ()  [unwired: 1 out]
        n120 = Close Reference(reference=w361, error in (no error)=w360) -> ()  [unwired: 1 out]
        n121 = Close Reference(reference=w338, error in (no error)=w337) -> ()  [unwired: 1 out]
        n122 = Close Reference(reference=w340, error in (no error)=w341) -> ()  [unwired: 1 out]
        n123 = Close Reference(reference=w343, error in (no error)=w344) -> ()  [unwired: 1 out]
        n124 = local read "Load Feedback"() -> (w369:dbl)
        n125 = Close Reference(reference=w349, error in (no error)=w348) -> ()  [unwired: 1 out]
        n126 = property class="Bool (strict)"(reference=w357, "DisabledEnum"=T2."Disabled and Grayed Out" ("Disabled")) -> (reference out=w355:refnum<vi>, error out=w356:errorcluster)  [unwired: 1 in]
        n127 = call <vilib>:"PID Autotuning.vi"("autotune? (F)"=w339, "reinitialize? (F)"=w335, "output range"=w350, "PID gains"=w358, "process variable"=w369, "setpoint"=w370) -> ("output"=w367:dbl)  [unwired: 2 in, 3 out]
        n128 = Subtract(x=w369, y=w370) -> (x-y=w374:dbl)
        n129 = Close Reference(reference=w355, error in (no error)=w356) -> ()  [unwired: 1 out]
        n130 = Less Or Equal?(x=w374, y=w346) -> (x <= y?=w373:bool)
        n131 = Absolute Value(x=w367) -> (abs(x)=w366:dbl)
        n132 = Unbundle By Name(w325) -> ("PID.actpid"=w329:refnum<vi>)
        n133 = Multiply(x=w366, y=w334) -> (x*y=w365:dbl)
        n134 = Subtract(x=w330, y=w365) -> (x-y=w364:dbl)
        n135 = Absolute Value(x=w364) -> (abs(x)=w326:dbl)
        n136 = property class="DigNum (strict)"(reference=w329, "Value"=w326) -> (reference out=w327:refnum<vi>, error out=w328:errorcluster)  [unwired: 1 in]
        n137 = In Range and Coerce(upper limit=2.0, x=w326, lower limit=0.1) -> (coerced(x)=w372:dbl)  [unwired: 1 out]
        n138 = Close Reference(reference=w327, error in (no error)=w328) -> ()  [unwired: 1 out]
        n139 = Greater Than 0?(x=w367) -> (x > 0?=w368:bool)
        n140 = flat-sequence {
          tunnel: w372 -> [w381]
          tunnel: [w381] -> w375
          tunnel: w325 -> [w377]
          frame #0 {
            n141 = Unbundle By Name(w377) -> ("PID.reinit 3"=w380:refnum<vi>)
            n142 = property class="Bool (strict)"(reference=w380, "Value"=FALSE) -> (reference out=w378:refnum<vi>, error out=w379:errorcluster)  [unwired: 1 in]
            n143 = Close Reference(reference=w378, error in (no error)=w379) -> ()  [unwired: 1 out]
          }
        }
        "Load" <- w370
        "apply load 2" <- TRUE ("apply load 2")
      }
    }
    n144 = case shown="True" w35 {
      tunnel: w4 -> [w230 w240]
      tunnel: w17 -> [_ w238]
      frame False {
        n145 = Unbundle By Name(w230) -> ("PID.pulses LoadDiff(11..50)"=w234:refnum<vi>)
        n146 = Unbundle By Name(w230) -> ("PID.pulses LoadDiff(11..50)"=w235:refnum<vi>)
        n147 = property class="DigNum (strict)"(reference=w234) -> (reference out=w232:refnum<vi>, error out=w233:errorcluster, "Value"=w231:dbl)  [unwired: 1 in]
        n148 = Close Reference(reference=w232, error in (no error)=w233) -> ()  [unwired: 1 out]
        n149 = property class="DigNum (strict)"(reference=w235, "Value"=w231) -> (reference out=w237:refnum<vi>, error out=w236:errorcluster)  [unwired: 1 in]
        n150 = Close Reference(reference=w237, error in (no error)=w236) -> ()  [unwired: 1 out]
      }
      frame True {
        n151 = Unbundle By Name(w240) -> ("PID.Ramp MulFac"=w247:refnum<vi>)
        n152 = property class="DigNum (strict)"(reference=w247) -> (reference out=w245:refnum<vi>, error out=w246:errorcluster, "Value"=w244:dbl)  [unwired: 1 in]
        n153 = Unbundle By Name(w240) -> ("PID.pulses LoadDiff(11..50)"=w241:refnum<vi>)
        n154 = Close Reference(reference=w245, error in (no error)=w246) -> ()  [unwired: 1 out]
        n155 = Multiply(x=w238, y=w244) -> (x*y=w239:dbl)
        n156 = property class="DigNum (strict)"(reference=w241, "Value"=w239) -> (reference out=w243:refnum<vi>, error out=w242:errorcluster)  [unwired: 1 in]
        n157 = Close Reference(reference=w243, error in (no error)=w242) -> ()  [unwired: 1 out]
      }
    }
    n158 = Unbundle By Name(w4) -> ("PID.pulses LoadDiff(2..10)"=w53:refnum<vi>)
    n159 = property class="DigNum (strict)"(reference=w103, "Value"=w102) -> (reference out=w105:refnum<vi>, error out=w104:errorcluster)  [unwired: 1 in]
    n160 = property class="Ring (strict)"(reference=w29) -> (reference out=w30:refnum<vi>, error out=w28:errorcluster, "Value"=w27:u16)  [unwired: 1 in]
    n161 = property class="DigNum (strict)"(reference=w45, "Value"=w42) -> (reference out=w43:refnum<vi>, error out=w44:errorcluster)  [unwired: 1 in]
    n162 = local read "Load Feedback"() -> (w162:dbl)
    n163 = local read "Load Feedback"() -> (w149:dbl)
    n164 = case shown="True" w127 {
      tunnel: [FALSE w186] -> w135
      tunnel: w11 -> [_ w185]
      frame False {
      }
      frame True {
        n165 = Less Or Equal?(x=w185, y=0.9) -> (x <= y?=w186:bool)
      }
    }
    n166 = local read "Set Load 2"() -> (w152:dbl)
    n167 = Divide(x=w42, y=100.0) -> (x/y=w150:dbl)
    n168 = Close Reference(reference=w30, error in (no error)=w28) -> ()  [unwired: 1 out]
    n169 = property class="DigNum (strict)"(reference=w53) -> (reference out=w51:refnum<vi>, error out=w52:errorcluster, "Value"=w50:dbl)  [unwired: 1 in]
    n170 = Close Reference(reference=w105, error in (no error)=w104) -> ()  [unwired: 1 out]
    n171 = Equal?(x=w27, y=w141) -> (x = y?=w136:bool)
    n172 = case shown="False" w137 {
      tunnel: [w217 w219] -> w144
      tunnel: w129 -> [w218 _]
      tunnel: w46 -> [_ w219]
      tunnel: w2 -> [w215 _]
      frame False {
        n173 = Select(t=6.0, s=w218, f=w215) -> (s? t:f=w217:dbl)
      }
      frame True {
      }
    }
    n174 = Subtract(x=w133, y=w162) -> (x-y=w160:dbl)
    n175 = Close Reference(reference=w43, error in (no error)=w44) -> ()  [unwired: 1 out]
    n176 = case shown="False" w137 {
      tunnel: w133 -> [w249 _]
      tunnel: [w248 1.0 ("y")] -> w142
      frame False {
        n177 = case shown="0..5, Default" w249 {
          tunnel: [0.1 ("y") 3.0 ("y")] -> w248
          frame 0..5, Default {
          }
          frame 6.. {
          }
        }
      }
      frame True {
      }
    }
    n178 = local read "Load Feedback"() -> (w177:dbl)
    n179 = Subtract(x=w152, y=w149) -> (x-y=w166:dbl)
    n180 = Multiply(x=w152, y=w150) -> (x*y=w148:dbl)
    n181 = local read "Load"() -> (w176:dbl)
    n182 = Absolute Value(x=w160) -> (abs(x)=w161:dbl)
    n183 = Close Reference(reference=w51, error in (no error)=w52) -> ()  [unwired: 1 out]
    n184 = Subtract(x=w176, y=w177) -> (x-y=w175:dbl)
    n185 = Absolute Value(x=w175) -> (abs(x)=w174:dbl)
    n186 = Less Or Equal?(x=w161, y=w142) -> (x <= y?=w155:bool)
    n187 = Absolute Value(x=w166) -> (abs(x)=w165:dbl)
    n188 = case shown="0, 1" w174 {
      tunnel: [w268 w275 w285 20.0 ("f") 20.0 ("f") 20.0 ("f") 30.0 ("f") 50.0 ("f")] -> w62
      tunnel: w136 -> [_ w274 _ _ _ _ _ _]
      tunnel: w129 -> [w270 w273 _ _ _ _ _ _]
      tunnel: w4 -> [_ w272 w286 _ _ _ _ _]
      tunnel: w50 -> [_ w271 _ _ _ _ _ _]
      frame 0, 1 {
        n189 = Select(t=3.0 ("f"), s=w270, f=1.0) -> (s? t:f=w268:dbl)
      }
      frame 2..10, Default {
        n190 = case shown="True" w274 {
          tunnel: [w277 w280] -> w275
          tunnel: w273 -> [w278 _]
          tunnel: w272 -> [_ w281]
          tunnel: w271 -> [w276 _]
          frame False {
            n191 = Select(t=9.0 ("f"), s=w278, f=w276) -> (s? t:f=w277:dbl)
          }
          frame True {
            n192 = Unbundle By Name(w281) -> ("PID.pulses LoadDiff(2..10)"=w282:refnum<vi>)
            n193 = property class="DigNum (strict)"(reference=w282) -> (reference out=w284:refnum<vi>, error out=w283:errorcluster, "Value"=w280:dbl)  [unwired: 1 in]
            n194 = Close Reference(reference=w284, error in (no error)=w283) -> ()  [unwired: 1 out]
          }
        }
      }
      frame 11..50 {
        n195 = Unbundle By Name(w286) -> ("PID.pulses LoadDiff(11..50)"=w288:refnum<vi>)
        n196 = property class="DigNum (strict)"(reference=w288) -> (reference out=w287:refnum<vi>, error out=w289:errorcluster, "Value"=w285:dbl)  [unwired: 1 in]
        n197 = Close Reference(reference=w287, error in (no error)=w289) -> ()  [unwired: 1 out]
      }
      frame 51..80 {
      }
      frame 81..100 {
      }
      frame 101..150 {
      }
      frame 151..500 {
      }
      frame 501..12000 {
      }
    }
    n198 = Less Or Equal?(x=w165, y=w148) -> (x <= y?=w163:bool)
    n199 = case shown="False" w135 {
      tunnel: w4 -> [w200 w208]
      frame False {
        n200 = Unbundle By Name(w200) -> ("PID.PulseControlRamp(diff<=3N)"=w201:refnum<vi>)
        n201 = Unbundle By Name(w200) -> ("PID.pulses LoadDiffRamp(2..10)"=w206:refnum<vi>)
        n202 = property class="DigNum (strict)"(reference=w206, "Value"=9.0 ("pulses LoadDiffRamp(2..10)")) -> (reference out=w204:refnum<vi>, error out=w205:errorcluster)  [unwired: 1 in]
        n203 = property class="DigNum (strict)"(reference=w201, "Value"=3.0 ("pulses LoadDiffRamp(2..10)")) -> (reference out=w198:refnum<vi>, error out=w202:errorcluster)  [unwired: 1 in]
        n204 = Close Reference(reference=w204, error in (no error)=w205) -> ()  [unwired: 1 out]
        n205 = Close Reference(reference=w198, error in (no error)=w202) -> ()  [unwired: 1 out]
      }
      frame True {
        w209 = 1.0 ("pulses LoadDiffRamp(2..10)")
        n206 = Unbundle By Name(w208) -> ("PID.PulseControlRamp(diff<=3N)"=w210:refnum<vi>)
        n207 = Unbundle By Name(w208) -> ("PID.pulses LoadDiffRamp(2..10)"=w214:refnum<vi>)
        n208 = property class="DigNum (strict)"(reference=w214, "Value"=w209) -> (reference out=w212:refnum<vi>, error out=w213:errorcluster)  [unwired: 1 in]
        n209 = property class="DigNum (strict)"(reference=w210, "Value"=w209) -> (reference out=w207:refnum<vi>, error out=w211:errorcluster)  [unwired: 1 in]
        n210 = Close Reference(reference=w212, error in (no error)=w213) -> ()  [unwired: 1 out]
        n211 = Close Reference(reference=w207, error in (no error)=w211) -> ()  [unwired: 1 out]
      }
    }
    n212 = Unbundle By Name(w4) -> ("PID.pulses"=w57:refnum<vi>)
    n213 = Unbundle By Name(w4) -> ("PID.pulsesSent"=w65:refnum<vi>)
    n214 = Unbundle By Name(w4) -> ("Main Screen.NLt"=w61:refnum<vi>)
    n215 = property class="DigNum (strict)"(reference=w65, "Value"=w62) -> (reference out=w63:refnum<vi>, error out=w64:errorcluster)  [unwired: 1 in]
    n216 = Select(t=w144, s=w155, f=w62) -> (s? t:f=w54:dbl)
    n217 = Close Reference(reference=w63, error in (no error)=w64) -> ()  [unwired: 1 out]
    n218 = property class="DigNum (strict)"(reference=w57, "Value"=w54) -> (reference out=w55:refnum<vi>, error out=w56:errorcluster)  [unwired: 1 in]
    n219 = Unbundle By Name(w4) -> ("PID.apply load"=w93:refnum<vi>)
    n220 = Unbundle By Name(w4) -> ("Main Screen.Load En"=w88:refnum<vi>)
    n221 = Close Reference(reference=w55, error in (no error)=w56) -> ()  [unwired: 1 out]
    n222 = Not(x=w163) -> (.not. x?=w147:bool)
    n223 = property class="Bool (strict)"(reference=w93) -> (reference out=w91:refnum<vi>, error out=w92:errorcluster, "Value"=w87:bool)  [unwired: 1 in]
    n224 = property class="Bool (strict)"(reference=w88) -> (reference out=w90:refnum<vi>, error out=w89:errorcluster, "Value"=w86:bool)  [unwired: 1 in]
    n225 = Wait (ms)(milliseconds to wait=u32 1) -> ()  [unwired: 1 out]
    n226 = Unbundle By Name(w4) -> ("Platform Settings.Heave COM Status"=w10:refnum<vi>)
    n227 = Close Reference(reference=w91, error in (no error)=w92) -> ()  [unwired: 1 out]
    n228 = Close Reference(reference=w90, error in (no error)=w89) -> ()  [unwired: 1 out]
    n229 = Or(x=w87, y=w86) -> (x .or. y?=w173:bool)
    n230 = property class="Bool (strict)"(reference=w10) -> (reference out=w8:refnum<vi>, error out=w9:errorcluster, "Value"=w7:bool)  [unwired: 1 in]
    n231 = Close Reference(reference=w8, error in (no error)=w9) -> ()  [unwired: 1 out]
    n232 = call "Elapsed Time2"("Time Target (s)"=w154) -> ("Time has Elapsed"=w178:bool)  [unwired: 11 in, 7 out]
    n233 = local read "Set Load 2"() -> (w167:dbl)
    n234 = And(x=w178, y=w173) -> (x .and. y?=w172:bool)
    n235 = Not(x=w7) -> (.not. x?=w153:bool)
    n236 = Greater Than 0?(x=w167) -> (x > 0?=w171:bool)
    n237 = And(x=w172, y=w153) -> (x .and. y?=w139:bool)
    n238 = Bundle("Value"=w159, "Load Feedback"=w138, "output"=w158) -> (w157:T4)  [unwired: 1 in]
    n239 = case shown="True" w139 {
      tunnel: w157 -> [_ w262]
      tunnel: w4 -> [_ w263]
      frame False {
      }
      frame True {
        n240 = Unbundle By Name(w263) -> ("PID.gFF Rot"=w266:refnum<vi>)
        n241 = property class="WFChart (strict)"(reference=w266, "Value"=w262) -> (reference out=w264:refnum<vi>, error out=w265:errorcluster)  [unwired: 1 in]
        n242 = Close Reference(reference=w264, error in (no error)=w265) -> ()  [unwired: 1 out]
      }
    }
    n243 = And(x=w139, y=w171) -> (x .and. y?=w164:bool)
    n244 = Select(t=w182, s=w170, f="-" ("direction")) -> (s? t:f=w180:string)
    n245 = Absolute Value(x=w154) -> (abs(x)=w169:dbl)
    n246 = call <vilib>:"Trim Whitespace.vi"("string"=w180) -> ("trimmed string"=w168:string)  [unwired: 1 in]
    n247 = And(x=w164, y=w147) -> (x .and. y?=w58:bool)
    n248 = case shown="True" w58 {
      tunnel: w168 -> [_ w300]
      tunnel: w169 -> [_ _]
      tunnel: w54 -> [_ w299]
      frame False {
      }
      frame True {
        n249 = Number To Decimal String(number=w299) -> (decimal integer string=w298:string)  [unwired: 1 in]
        n250 = local read "WriteCC1"() -> (w295:string[])
        n251 = Concatenate Strings("Z;", w300, w298) -> (w297:string)
        n252 = Insert Into Array(array=w295, new element=w297) -> (w296:string[])  [unwired: 1 in]
        n253 = local write "WriteCC1"(w296) -> ()
      }
    }
    n254 = property class="Bool (strict)"(reference=w61, "Value"=w58) -> (reference out=w59:refnum<vi>, error out=w60:errorcluster)  [unwired: 1 in]
    n255 = Close Reference(reference=w59, error in (no error)=w60) -> ()  [unwired: 1 out]
    "Motorised Loading Loop" <- w156
  }
